vi "_시리얼_Mark10-헤드이동.vi"(4 "동작 모드":string(combo)="STOP", 5 "시리얼 포트":refnum<visa-resource-name>="COM5") -> (2 "VISA 리소스 이름 출력":refnum<visa-resource-name>)   [LabVIEW 2015]
panel:
  # "MARK10 헤드 이동 제어"
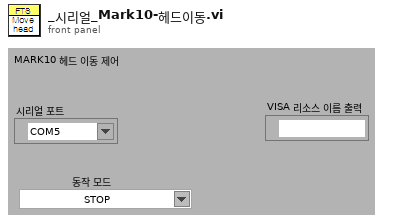
[diagram p1: front panel]
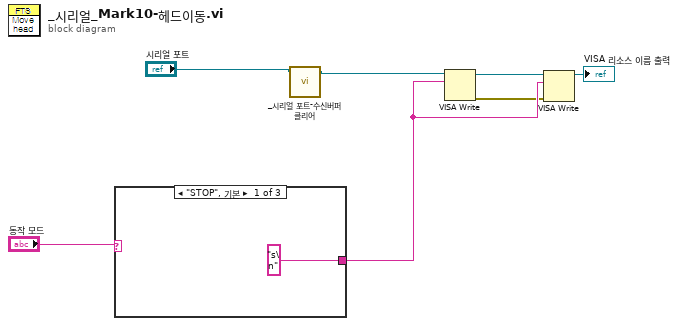
[diagram p0: block diagram]
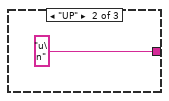
[diagram p2: hidden frame]
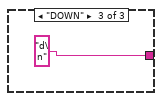
[diagram p3: hidden frame]
diagram:
  n1 = case shown="\"STOP\", 기본" "동작 모드" {
    tunnel: ["s\n" "u\n" "d\n"] -> w5
    frame "STOP", Default {
    }
    frame "UP" {
    }
    frame "DOWN" {
    }
  }
  n2 = call "_시리얼 포트-수신버퍼 클리어.vi"("시리얼 포트"="시리얼 포트") -> ("시리얼 포트 out"=w1:refnum<visa-resource-name>)  [unwired: 3 in, 1 out]
  n3 = VISA Write(VISA resource name=w1, write buffer=w5) -> (VISA resource name out=w6:refnum<visa-resource-name>, error out=w4:errorcluster)  [unwired: 1 in, 1 out]
  n4 = VISA Write(VISA resource name=w6, write buffer=w5, error in (no error)=w4) -> (VISA resource name out=→"VISA 리소스 이름 출력":refnum<visa-resource-name>)  [unwired: 2 out]
